vi "Write Comp Driver Tuning.vi"(8 "error in (no error)":errorcluster, 10 "Comp Driver Tuning":T1, 11 "Comp Driver in":refnum<class "Comp Driver.lvclass">) -> (0 "error out":errorcluster, 3 "Comp Driver out":refnum<class "Comp Driver.lvclass">)   [LabVIEW 2014, in "Comp Driver.lvlib" / "Comp Driver.lvclass"]
uses:
  Comp Driver.lvclass
  Comp Driver Tuning.ctl
  Comp Driver.lvclass/Comp Driver.ctl
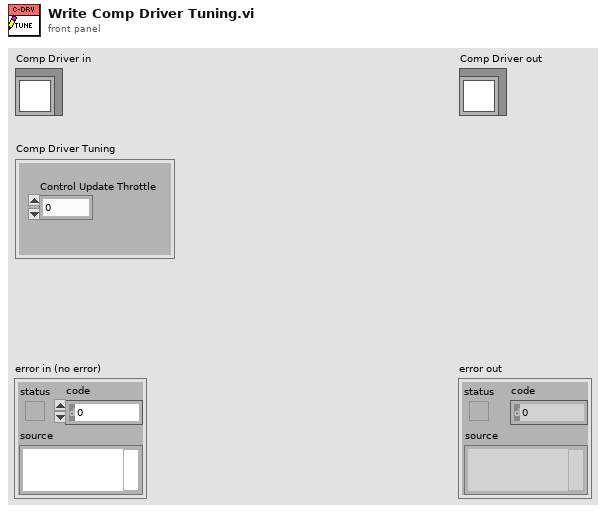
[diagram p1: front panel]
types:
  T1 = typedef "Comp Driver.lvlib/Comp Driver.lvclass/Comp Driver Tuning.ctl" = cluster{"Control Update Throttle":u32}
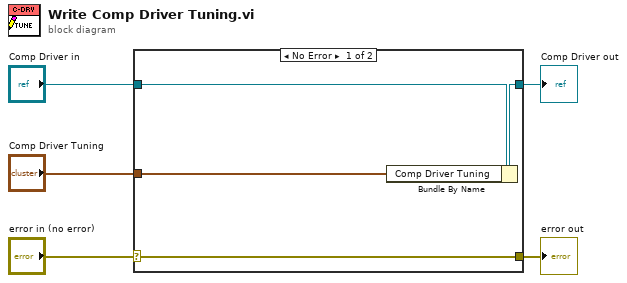
[diagram p0: block diagram]
diagram:
  n1 = case shown="No Error" "error in (no error)" {
    selector: "error in (no error)" -> [w9 w10]
    tunnel: [w9 w10] -> w4
    tunnel: [w7 w11] -> w2
    tunnel: "Comp Driver in" -> [w8 w11]
    tunnel: "Comp Driver Tuning" -> [w6 _]
    frame No Error {
      n2 = Bundle By Name(cluster=w8, "Comp Driver Tuning"=w6) -> (w7:refnum<class "Comp Driver.lvclass">)
    }
    frame Error {
    }
  }
  "error out" <- w4
  "Comp Driver out" <- w2
